vi "Prompt.vi"(11 "URL":string caption="Go to this URL then press Authorize") -> (0 "error out":errorcluster, 3 "verifier":string)   [LabVIEW 2012]
panel:
  in  "URL 2":string caption="Enter Verifier here"
  in  "stop":bool
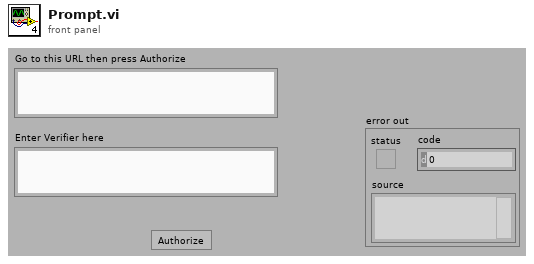
[diagram p1: front panel]
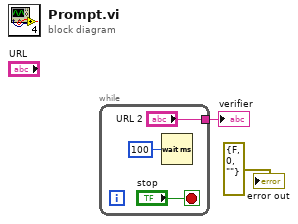
[diagram p0: block diagram]
diagram:
  n1 = while {
    tunnel: ["URL 2"] -> w1
    stop <- "stop" stop-if-true
    n2 = Wait (ms)(milliseconds to wait=u32 100) -> ()  [unwired: 1 out]
  }
  "verifier" <- w1
  "error out" <- errorcluster {"status"=FALSE, "code"=0, "source"=""} ("error out")
